vi "IMUOpen.vi"(4 "MagCal":bool=TRUE, 5 "Accel Set":T4={"Data Rate"=enum."1.344 kHz", "Range"=0, "HPF Enable"=FALSE, "HPCF"=enum."00", "Sense Enable"=TRUE, "Accel Scale"={"Xscale"=1.0, "Yscale"=1.0, "Zscale"=1.0}, "Motion Thresh"=0.0} {"Range" items=["+/- 2 G", "+/- 4 G", "+/- 8 G", "+/- 16 G"]}, 6 "Mag Set":T2={"Data Rate"=enum."220 Hz", "Range"=1, "Sense Enable"=TRUE, "Mag Scale"={"Xscale"=1.0, "Yscale"=1.0, "Zscale"=1.0}, "Mag Offset"={"Xzero"=0.0, "Yzero"=0.0, "Zzero"=0.0}, "Anomaly Thresh"=0.0, "Local Mag"=0.0} {"Range" items=["+/- 130 uT"=1, "+/- 190 uT"=2, "+/- 250 uT"=3, "+/- 400 uT"=4, "+/- 470 uT"=5, "+/- 560 uT"=6, "+/- 810 uT"=7]}, 7 "Gyro Set":T5={"Data Rate"=enum."800 Hz", "Range"=0, "HPF Enable"=FALSE, "HPCF"=enum."0000", "Sense Enable"=TRUE} {"Range" items=["+/- 245 deg/sec", "+/- 500 deg/sec", "+/- 2000 deg/sec"]}, 8 "error in (no error)":errorcluster, 9 "Fast":bool=TRUE, 10 "CalSamples":i32=60, 11 "I2C Bus":T3) -> (0 "error out":errorcluster, 2 "Cal Result":T1, 3 "AdaIMUDevRef Out":T6={"DevStatus"={"status"=FALSE, "code"=0, "source"=""}, "Gyro Address"=0, "Gyro Range"=0, "Mean Rates"={"Xmo"=0.0, "Ymo"=0.0, "Zmo"=0.0}, "StdDev Rates"={"Xsdo"=0.0, "Ysdo"=0.0, "Zsdo"=0.0}, "Fast"=FALSE, "Reset"=FALSE, "Accel Address"=0, "Accel Range"=0, "Accel Scale"={"Xscale"=0.0, "Yscale"=0.0, "Zscale"=0.0}, "Mag Address"=0, "Mag Range"=0, "G Sense"=FALSE, "A Sense"=FALSE, "M Sense"=FALSE, "Accel Offset"={"Xzero"=0.0, "Yzero"=0.0, "Zzero"=0.0}, "Motion Thresh"=0.0, "Mag Scale"={"Xscale"=1.0, "Yscale"=1.0, "Zscale"=1.0}, "Mag Offset"={"Xzero"=1.0, "Yzero"=1.0, "Zzero"=1.0}, "I2C Bus"=enum."I2C On-Board", "Handle"=0, "Anomaly Thresh"=0.0, "Local Mag"=0.0})   [LabVIEW 2015]
uses:
  IMUDevRef.ctl
  <vilib>/Rock Robotics/SystemInterfaces/i2clib/i2c_bus.ctl
  <vilib>/Platform/TimedLoop/XDataNode/timing_clust.ctl
  <vilib>/Platform/TimedLoop/XDataNode/nitl_modes.ctl
  <vilib>/Platform/TimedLoop/XDataNode/wakeup.ctl
  <vilib>/Utility/file.llb/Write To Spreadsheet File (DBL).vi
  <vilib>/platform/TimedLoop/XDataNode/XDataNode.xnode
  <vilib>/Platform/TimedLoop/XDataNode/XDNodeRunTimeDep.lvlib
  <vilib>/Analysis/NI_AALBase.lvlib
panel:
  in  "Mag Set 2":T2={"Data Rate"=enum."220 Hz", "Range"=1, "Sense Enable"=TRUE, "Mag Scale"={"Xscale"=1.0, "Yscale"=1.0, "Zscale"=1.0}, "Mag Offset"={"Xzero"=0.0, "Yzero"=0.0, "Zzero"=0.0}, "Anomaly Thresh"=0.0, "Local Mag"=0.0} {"Range" items=["+/- 130 uT"=1, "+/- 190 uT"=2, "+/- 250 uT"=3, "+/- 400 uT"=4, "+/- 470 uT"=5, "+/- 560 uT"=6, "+/- 810 uT"=7]}
  out "XY Mag, Cal'd":cluster{dbl[], dbl[]}(graph)
  out "Anomaly Tol (uT)":dbl
  out "Local Magnitude (uT)":dbl
  out "Mid-Pnt":dbl
  out "Half-Range":dbl
  out "Late?":bool
  in  "Period":i64=20
  out "Yaw":dbl(knob) scale=-180.0..180.0
  out "Pitch":dbl(knob) scale=-90.0..90.0
  out "Roll":dbl(knob) scale=-180.0..180.0
  in  "Reset":bool
  in  "Accel Set 2":T4={"Data Rate"=enum."1.344 kHz", "Range"=0, "HPF Enable"=FALSE, "HPCF"=enum."00", "Sense Enable"=TRUE, "Accel Scale"={"Xscale"=0.9852, "Yscale"=1.0101, "Zscale"=1.0101}, "Motion Thresh"=0.04} {"Range" items=["+/- 2 G", "+/- 4 G", "+/- 8 G", "+/- 16 G"]}
  in  "Gyro Set 2":T5={"Data Rate"=enum."800 Hz", "Range"=0, "HPF Enable"=FALSE, "HPCF"=enum."0000", "Sense Enable"=TRUE} {"Range" items=["+/- 245 deg/sec", "+/- 500 deg/sec", "+/- 2000 deg/sec"]}
  out "Xmagscale":dbl
  out "Ymagscale":dbl
  out "Ymagzero":dbl
  out "Xmagzero":dbl
  out "XY Mag":cluster{dbl[], dbl[]}(graph)
  out "stop loop":bool
  # "EXAMPLE MAGNETOMETER CAL PLOT - FOR REFERENCE"
  # "Magnetometer Cal Results"
  # "Use LM as Local Mag,\nwhich should be NOAA\nHorizontal Mag Intensity.\nUse AT as minimum\nAnomaly Threshold."
  # "Magnetometer Calibration Data Result\n\nLook for a constant radius circle - if not, repeat calibration.\n\nMagnetometer measurement error is generally classified into two categories, Hard Iron and Soft Iron effects.  Only Hard Iron effects\nare compensated here, as they appear more dominate.  Soft Iron effect compensation is a future improvement.  Performance is\nadequate as long as sources of Soft Iron distortion (non-magnetized Iron, Nickle, and Cobalt) are kept away from sensor\n(or vice versa).  If an ellipse is displayed, there is Soft Iron magnetic field interference.  Ensure the cal plot has equally sized X and Y\naxis ranges prior to visually inspecting the cal plot and making an ellipse determination.  If Soft Iron is detected, either relocate the\nIMU or discover and remove the offending material.  Run all motors and other actuators to verify that the Yaw output of the\nComplementary Filter is not significantly affected.  If so, it may be possible to relocate the IMU or shield the motor with\nmu-metal or similar.  Do not shield the IMU!"
  # "Reserved for future use."
  # "These controls/indicators are non-operational / they are here as example documentation only."
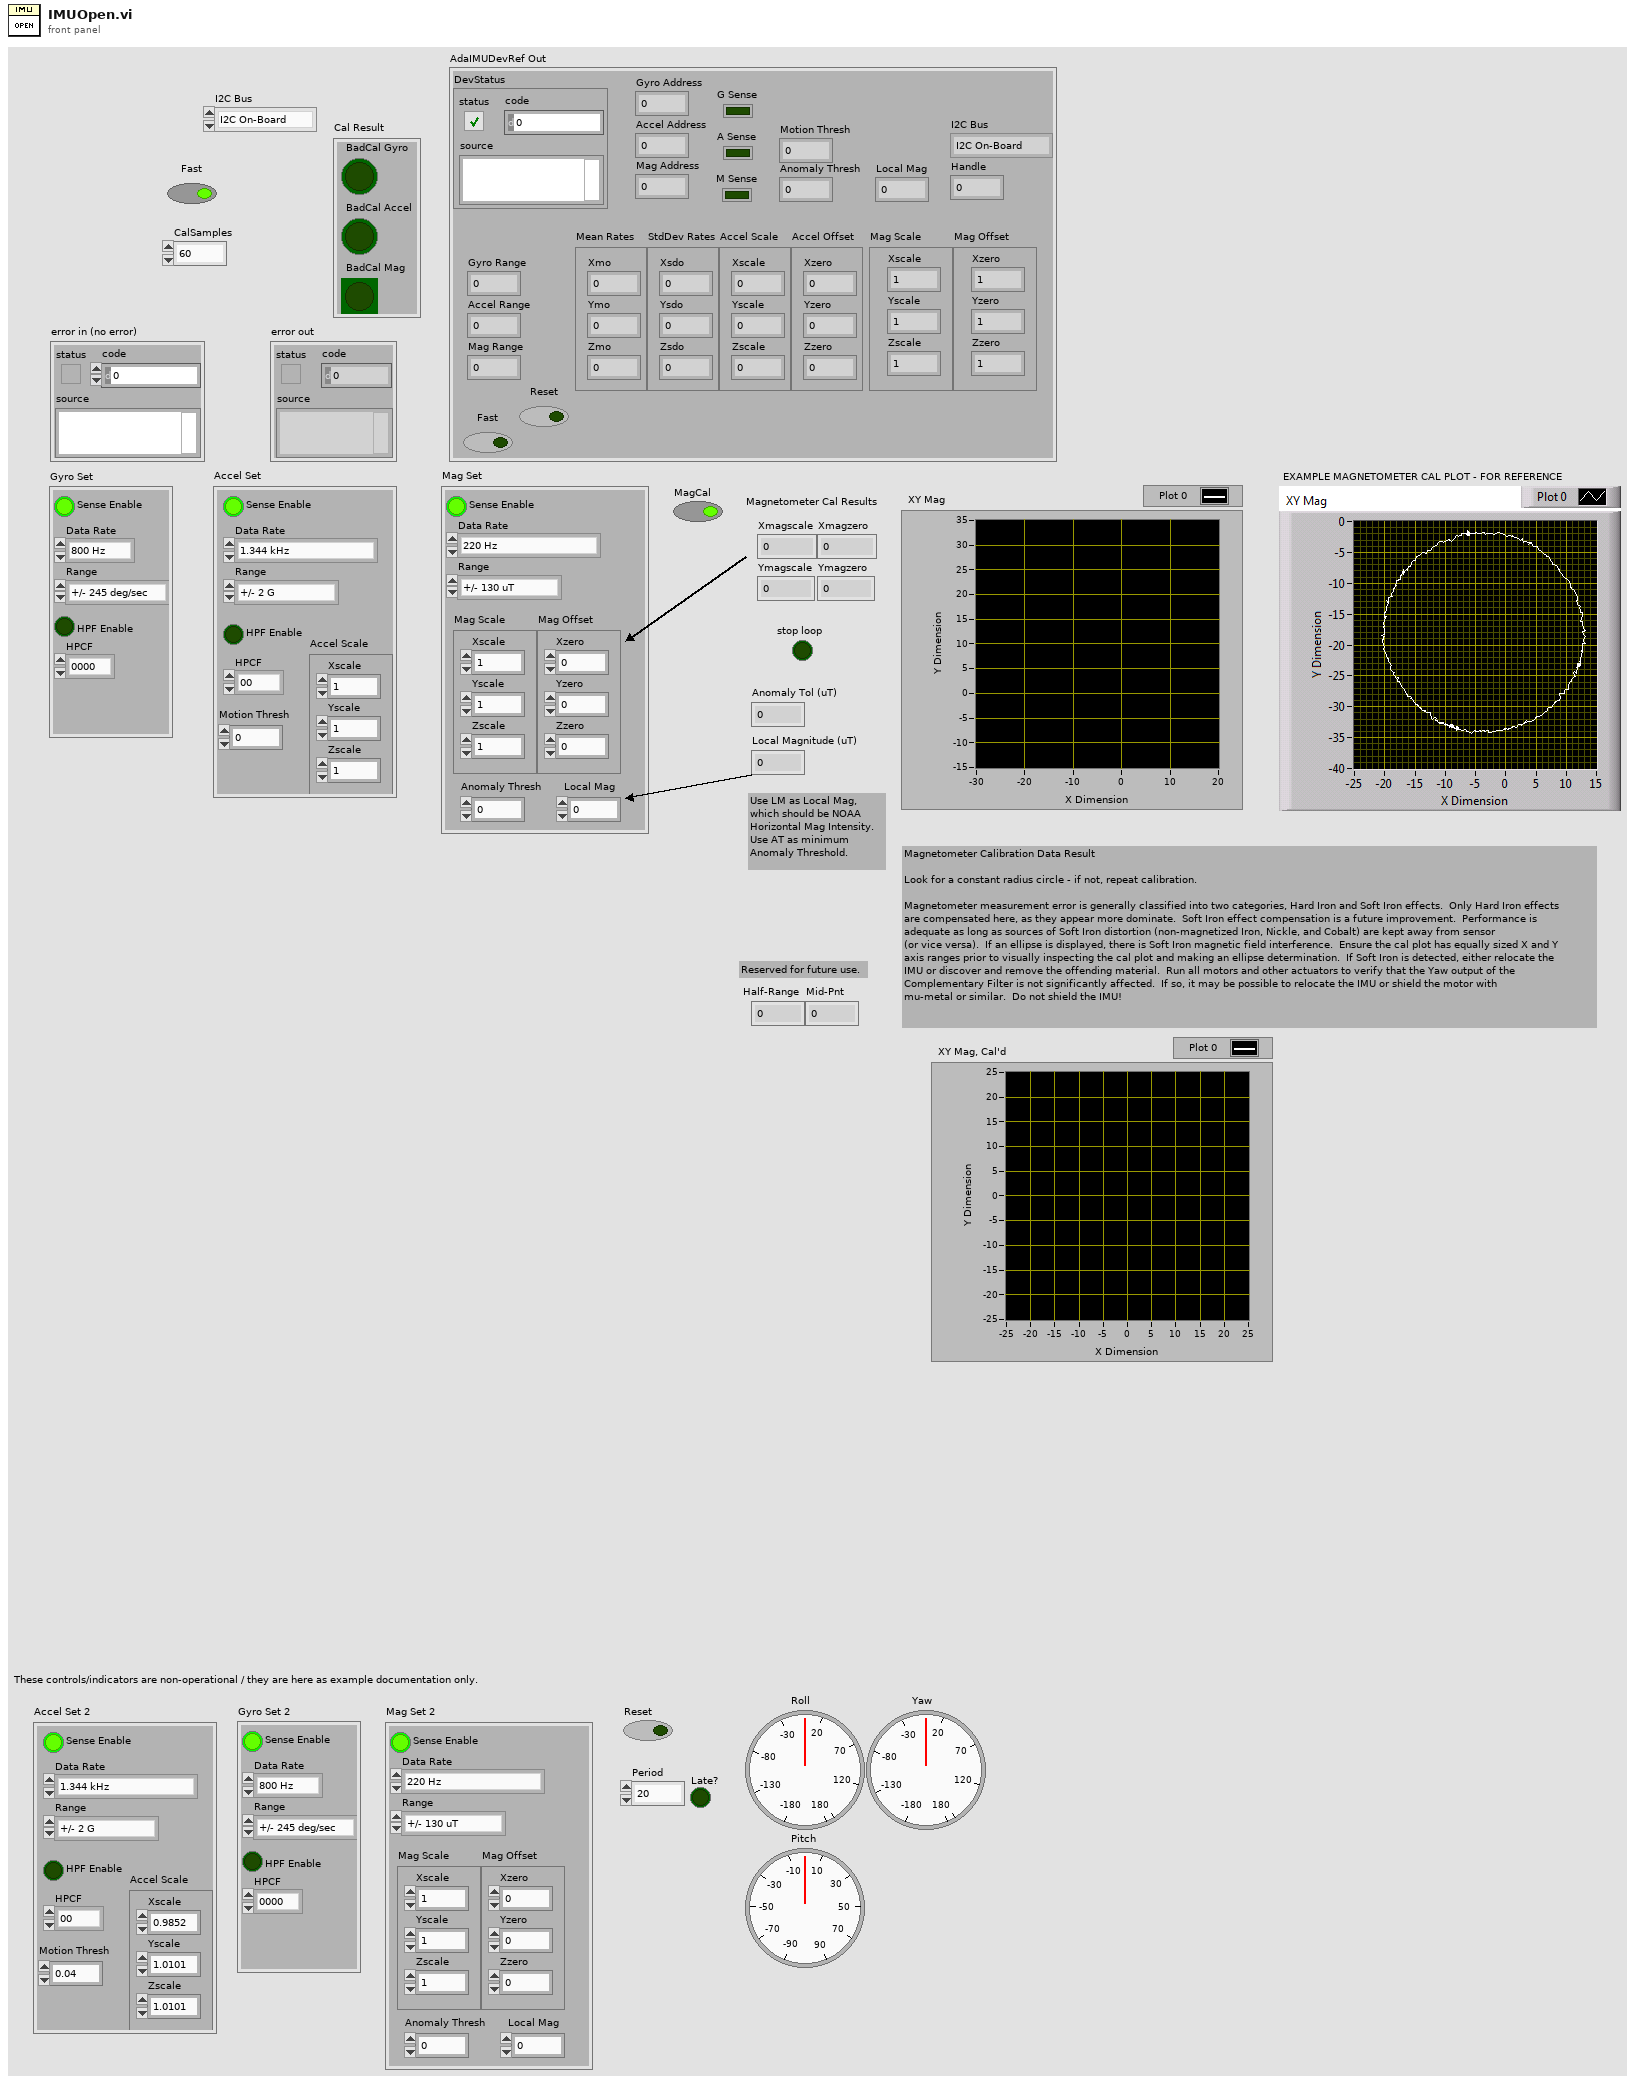
[diagram p1: front panel]
types:
  T1 = cluster{"BadCal Gyro":bool, "BadCal Accel":bool, "BadCal Mag":bool}
  T2 = cluster{"Data Rate":enum8{"0.75 Hz", "1.5 Hz", "3.0 Hz", "7.5 Hz", "15 Hz", "30 Hz", "75 Hz", "220 Hz"}, "Range":u8, "Sense Enable":bool, "Mag Scale":cluster{"Xscale":dbl, "Yscale":dbl, "Zscale":dbl}, "Mag Offset":cluster{"Xzero":dbl, "Yzero":dbl, "Zzero":dbl}, "Anomaly Thresh":dbl, "Local Mag":dbl}
  T3 = typedef "i2c_bus.ctl" = enum16{"I2C On-Board", "I2C MXP", "Invalid"}
  T4 = cluster{"Data Rate":enum8{"Power-down mode", "1 Hz", "10 Hz", "25 Hz", "50 Hz", "100 Hz", "200 Hz", "400 Hz", "Low-power mode only", "1.344 kHz"}, "Range":u8, "HPF Enable":bool, "HPCF":enum8{"00", "01", "10", "11"}, "Sense Enable":bool, "Accel Scale":cluster{"Xscale":dbl, "Yscale":dbl, "Zscale":dbl}, "Motion Thresh":dbl}
  T5 = cluster{"Data Rate":enum8{"100 Hz", "200 Hz", "400 Hz", "800 Hz"}, "Range":u8, "HPF Enable":bool, "HPCF":enum8{"0000", "0001", "0010", "0011", "0100", "0101", "0110", "0111", "1000", "1001"}, "Sense Enable":bool}
  T6 = typedef "IMUDevRef.ctl" = cluster{"DevStatus":errorcluster, "Gyro Address":u8, "Gyro Range":u8, "Mean Rates":cluster{"Xmo":dbl, "Ymo":dbl, "Zmo":dbl}, "StdDev Rates":cluster{"Xsdo":dbl, "Ysdo":dbl, "Zsdo":dbl}, "Fast":bool, "Reset":bool, "Accel Address":u8, "Accel Range":u8, "Accel Scale":cluster{"Xscale":dbl, "Yscale":dbl, "Zscale":dbl}, "Mag Address":u8, "Mag Range":u8, "G Sense":bool, "A Sense":bool, "M Sense":bool, "Accel Offset":cluster{"Xzero":dbl, "Yzero":dbl, "Zzero":dbl}, "Motion Thresh":dbl, "Mag Scale":cluster{"Xscale":dbl, "Yscale":dbl, "Zscale":dbl}, "Mag Offset":cluster{"Xzero":dbl, "Yzero":dbl, "Zzero":dbl}, "I2C Bus":T3, "Handle":i32, "Anomaly Thresh":dbl, "Local Mag":dbl}
  T7 = enum8{"0000", "0001", "0010", "0011", "0100", "0101", "0110", "0111", "1000", "1001"}
  T8 = typedef "WPI_I2CDevRef.ctl" = cluster{"DevStatus":errorcluster, "Device Address":u8, "Handle":i32, "I2C Bus":T3}
  T9 = typedef "XDNodeRunTimeDep.lvlib/timing_clust.ctl" = cluster{"Expected End [f-1]":u64, "Actual End [f-1]":u64, "Finished Late? [f-1]":bool, "Expected End [i-1]":u64, "Actual End [i-1]":u64, "Finished Late? [i-1]":bool, "Expected Start [i]":u64, "Actual Start [i]":u64, "Expected Start [f]":u64, "Actual Start [f]":u64, "Source Name":string, "Structure Name":string, "Period":i64, "Deadline":i64, "Offset":i64, "Start":i64, "Priority":i32, "Timeout":i32, "Mode":T10, "Wakeup Reason":T11, "Error":errorcluster, "Source Type":string, "Secondary Source Type":string, "Global End Time":u64, "Global Start Time":u64, "Frame Duration":u64, "Iteration Duration":u64, "Assigned CPU":i32, "I/O Scan Engine Mode":u32}
  T10 = typedef "XDNodeRunTimeDep.lvlib/nitl_modes.ctl" = enum32{"No Change", "Process missed periods, maintain original phase", "Discard missed periods, maintain original phase", "Process missed periods, ignore original phase", "Discard missed periods, ignore original phase"}
  T11 = typedef "XDNodeRunTimeDep.lvlib/wakeup.ctl" = enum32{"Normal", "Aborted", "Asynchronous wakeup", "Timing source error", "Timed loop error", "Timeout"}
  T12 = typedef "Gyro.ctl" = cluster{"Xrate":dbl, "Yrate":dbl, "Zrate":dbl, "Xdeg":dbl, "Ydeg":dbl, "Zdeg":dbl, "dt":dbl}
  T13 = typedef "Accel.ctl" = cluster{"Xaccel":dbl, "Yaccel":dbl, "Zaccel":dbl, "Motion":bool, "Threshold":dbl, "FreeFall":bool}
  T14 = typedef "Mag.ctl" = cluster{"Xmag":dbl, "Ymag":dbl, "Zmag":dbl, "Anomaly":bool}
  T15 = enum8{"Power-down mode", "1 Hz", "10 Hz", "25 Hz", "50 Hz", "100 Hz", "200 Hz", "400 Hz", "Low-power mode only", "1.344 kHz"}
  T16 = cluster{"Xscale":dbl, "Yscale":dbl, "Zscale":dbl}
  T17 = enum8{"0.75 Hz", "1.5 Hz", "3.0 Hz", "7.5 Hz", "15 Hz", "30 Hz", "75 Hz", "220 Hz"}
  T18 = cluster{"Accel Zero.Zzero":dbl, "Accel Zero.Zzero 2":dbl, "Accel Zero.Zzero 3":dbl}
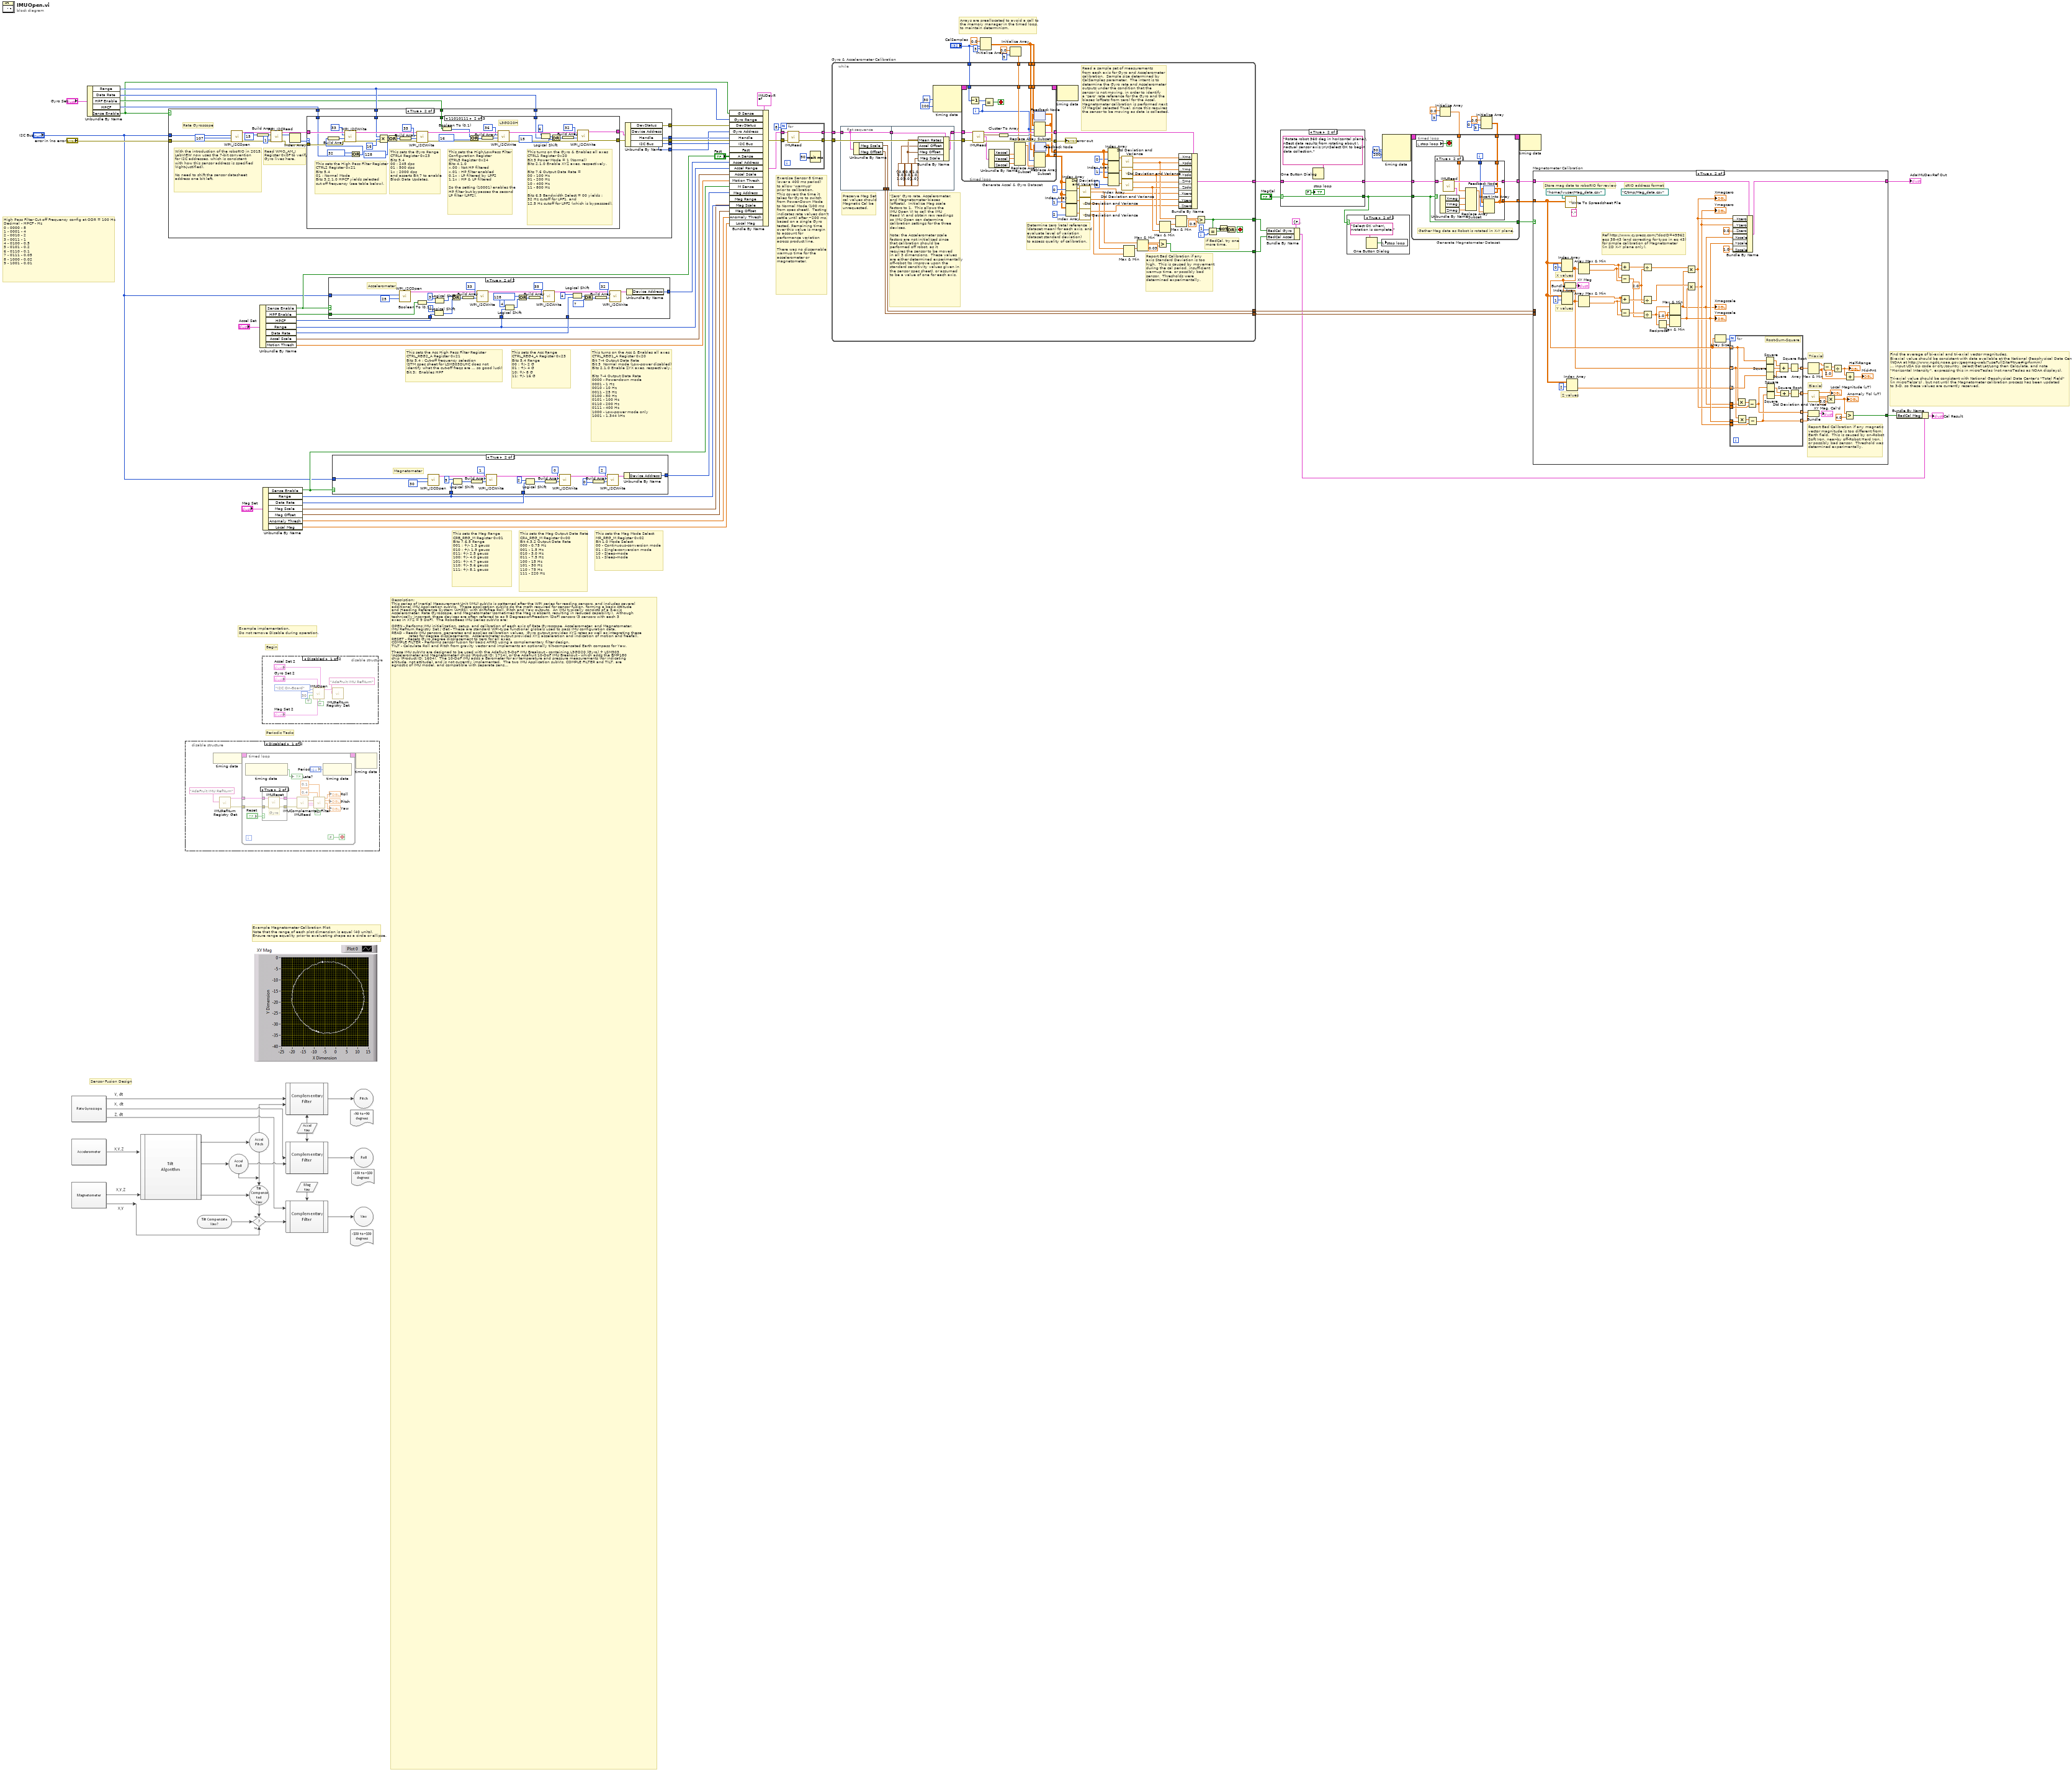
[diagram p0: block diagram]
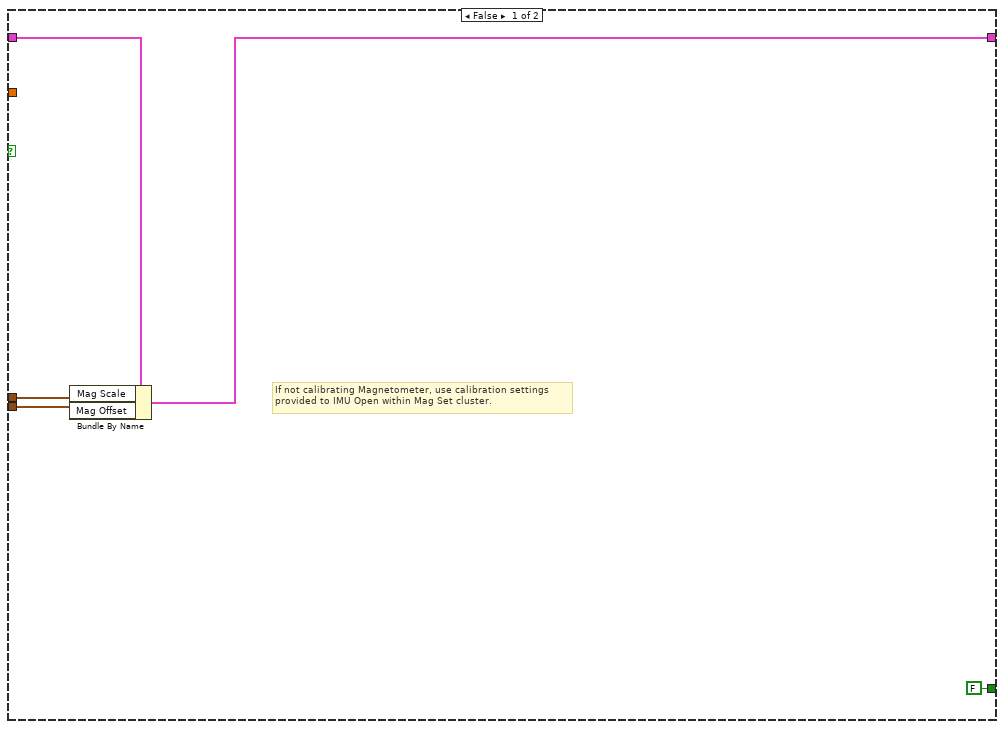
[diagram p2: hidden frame]
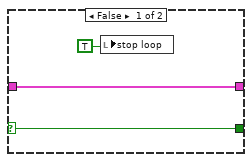
[diagram p5: hidden frame]
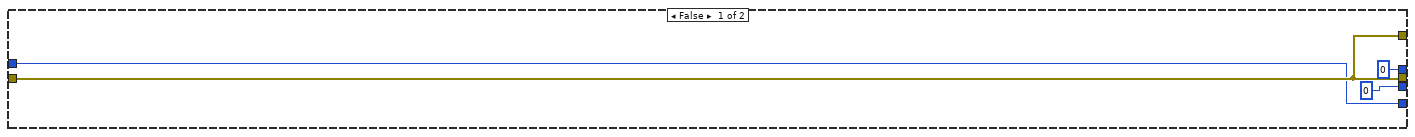
[diagram p9: hidden frame]
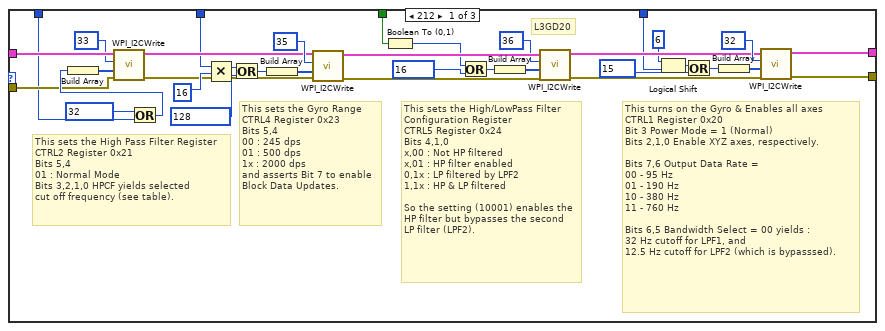
[diagram p10: hidden frame]
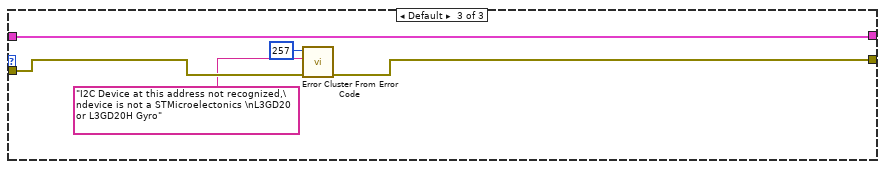
[diagram p11: hidden frame]
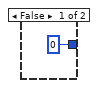
[diagram p12: hidden frame]
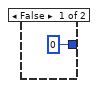
[diagram p13: hidden frame]
diagram:
  # "Find the average of bi-axial and tri-axial vector magnitudes.\nBi-axial value should be consistent with data available at the National Geophysical Data Center\n(NOAA at http://www.ngdc.noaa.gov/geomag-web/?useFullSite=true#igrfwmm)\n... input USA zip code or city/country, select Get Lat/Long then Calculate, and note\n\"Horizontal Intensity\", expressing this in microTeslas (not nanoTeslas as NOAA displays). \n\nTri-axial value should be consistent with National Geophysical Data Center's \"Total Field\"\n(in microTelsa's) , but not until the Magnetometer calibration process has been updated\nto 3-D, so these values are currently reserved."
  # "Arrays are preallocated to avoid a call to\nthe memory manager in the timed loop,\nto maintain determinism."
  # "Sensor Fusion Design"
  # "Example Magnetometer Calibration Plot\nNote that the range of each plot dimension is equal (40 units).\nEnsure range equality prior to evaluating shape as a circle or ellipse."
  # "Begin"
  # "Periodic Tasks"
  # "Example implementation.\nDo not remove Disable during operation."
  # "Description:\nThis series of Inertial Measurement Unit (IMU) subVIs is patterned after the WPI series for reading sensors, and includes several\nadditional IMU Application subVIs.  These application subVIs do the math required for sensor fusion, forming a basic Attitude\nand Heading Reference System (AHRS), with drift-free Roll, Pitch and Yaw outputs.  An IMU typically consists of a 3-axis \nAccelerometer, Rate Gyroscope, and Magnetometer (sometimes the Mag is absent, resulting in reduced capability).  Although\ntechnically incorrect, these devices are often referred to as 9 Degrees-of-Freedom (DoF) sensors (3 sensors with each 3\naxes in XYZ = 9 DoF).  The RoboBees IMU Series subVIs are:\n\nOPEN - Performs IMU initialization, setup, and calibration of each axis of Rate Gyroscope, Accelerometer, and Magnetometer.\nIMU RefNum Registry Set / Get - These are standard WPI-type functional globals used to pass IMU configuration data.\nREAD - Reads IMU sensors, generates and applies calibration values.  Gyro output provides XYZ rates as well as integrating these\n              rates for degree displacements.  Accelerometer output provides XYZ acceleration and indication of motion and freefall.\nRESET - Resets Gyro degree displacement to zero for all axes.\nCOMPLE FILTER - Performs sensor fusion for basic AHRS using a complementary filter design.\nTILT - Calculate Roll and Pitch from gravity vector and implements an optionally tilt-compensated Earth compass for Yaw.\n\nThese IMU subVIs are designed to be used with the Adafruit 9-DoF IMU Breakout - containing L3GD20 (Gyro) + LSM303 \n(Accelerometer and Magnetometer) chips (Product ID: 1714), or the Adafruit 10-DoF IMU Breakout - which adds the BMP180\nchip (Product ID: 1604).  The 10-DoF IMU adds a Barometer for air temperature and pressure measurements (for indicating\naltitude, not attitude), and is not currently implemented.  The two IMU Application subVIs, COMPLE FILTER and TILT, are\nagnostic of IMU model, and compatible with separate sensors, as long as all sensor axes are aligned properly.\n\nThe motivation to fusing these sensors is to combine their best properties and mitigate the worst properties of each.  The overall\nsensor fusion design is provided (to lower left) in block diagram form.  A major benefit is effective elimination of the drift inherent\nin the Rate Gyro when used alone.\n\nDesign:\nThe IMU OPEN subVI sets up each sensor based on the respective Set Cluster settings.  This includes setting the sensor range, output\ndata rate, enabling the High Pass Filter (Gyro and Accelerometer only), and selecting a High Pass Cut off Frequency.  Each sensor\ncan also be selectively enabled/disabled.  All sensors (except the Barometer), need to be enabled for a fully functional AHRS.  The\nIMU breakout board from Adafruit.com places all sensors on a common I2C bus for communication.  The sensor chip's I2C\nAddresses (in hex) and respective data sheets for I2C register references are:\n\nChip                      -  Sensor                - I2C Address  -  Data Sheet Reference\nLSM303DLHC      - Accelerometer   - 0x19               -  http://www.adafruit.com/datasheets/LSM303DLHC.PDF\nLSM303DLHC      - Magnetometer  - 0x1E               -  see above\nL3GD20(H)           - Rate Gyroscope - 0x6B               -  http://www.st.com/st-web-ui/static/active/en/resource/technical/document/\n                                                                                          datasheet/DM00036465.pdf\nBMP180               - Barometer           - 0x77               -  http://www.adafruit.com/datasheets/BST-BMP180-DS000-09.pdf\n\nNote: Adafruit modified both breakout board configurations in Oct of 2014 to upgrade the Gyro sensor from L3GD20 to L3GD20H\n(improved performance specifications).  This code should be compatible with each Gyro variant.  Guidance on the Gyro startup\nsequence is given in section 3.1 of ST MicroElectronics App Note AN4506 for L3GD20H : \nhttp://www.st.com/web/en/resource/technical/document/application_note/DM00119037.pdf\n\nAfter the sensors are set up, enabled sensors are turned on, IMU configuration data is loaded into an IMU Cluster, and sensor\ncalibration begins.\n\nCalibration:\nRaw readings from an IMU are not very useful until they are conditioned by carefully determined calibration parameters.\nSince reading the digital sensor values is a bit complicated, the IMU READ subVI is simply called by IMU OPEN to produce the raw\nmeasurement values used to characterize the sensor.  The calibration is only good for the range selected during the cal process.\n\nThe calibration process used here is determining the values 'm' and 'b' for the assumed linear sensor model Y=mX+b for each\nparameter/axis pair, where 'X' is the raw sensor reading, 'm' and 'b' are cal parameters, and 'Y' is the corrected sensor reading.\nThe sensor is 'exercised' eight times to allow the Gyro readings to reach steady-state, which improves the calibration.  With the\ndefault cal sample size of 60, the Gyro/Accelerometer cal process takes about 2.2 seconds, which is about 0.2 seconds longer\nthan the default cal time for the OPEN subVI for an analog Gyro.   The Gyro and Accelerometer cal is performed first\n(simultaneously), and the robot needs to be completely still during this time (as is required with an analog Gyro).  Since the cal\nis conducted within the OPEN subVI, and OPEN is generally placed in Begin (in FIRST Robotics) before the robot can move itself,\nthis requirement is easily fulfilled.  Care, however, must still be taken to ensure no external bumps occur during this cal.  This\ncode can actually detect if a physical disturbance occurred, and recalibrate automatically as a mitigation (no extra charge).\n\nRecalling the model Y=mX+b, for the IMU Gyro, 'm' is taken from the spec sheet as the gain (sensitivity) for each axis.  Value 'b',\nwhich is bias from zero, is determined by taking the statistical mean of a sample of Gyro rate measurements while the sensor is still.\n\nFor the Accelerometer, 'm' should be determined off-robot, as it requires the sensor to be moved in all 3 dimensions.  These values\nare either determined experimentally off-robot (to improve upon the standard sensitivity values given in the sensor spec sheet), or\nassumed to be a value of one for each axis.  To determine experimentally, find the maximum and minimum values of each axis as\nthey are rotated (slowly) through vertical.  The axis sensitivity is half of the signed difference between max and min.  Value 'b' is\ndetermined automatically by taking the statistical mean of a sample of Accelerometer measurements while the sensor is still.\n\nThe fun really begins with the Magnetometer calibration.  Proper Mag cal requires the sensor to be rotated in all 3 dimensions, but\nunlike the Accelerometer, the Mag must be rotated with the rest of the robot to account for how the robot itself disturbs the Earth's\nmagnetic field (this is a lot easier when the Mag sensor is installed in a smart phone.).  Since one typically would not have available\na 3-axis non-ferrous robot gimbal, the cal process is designed to support a 2-D calibration in the X-Y (horizontal) plane only.\n\nIn another departure from the Gyro/Accel cal, sample data from the Mag must be taken as the robot is moving.  This process is\noptional to allow the 'm' and 'b' Mag cal parameters to be determined during final testing, and then loaded into the Mag Set Cluster\nfor operations (i.e. competition).  If selected, the Mag cal process first instructs you to begin rotating the robot (manually) with a \npop-up dialog box.  Selecting OK initiates data collection, and provides a second dialog box to allow you to signal when you've \ncompleted a 360 degree rotation.  \n\nOnce complete, the X and Y axis 'm' and 'b' parameters are calculated and displayed on the IMU OPEN Front Panel as 'scale' and\n'zero', respectively.  An XY graph of the data is also provided to allow visual inspection of the cal result - look for a nicely shaped\ncircle (see example at left), if not, repeat the cal.  If you like the plot, load the X and Y axis scale and zero parameters into the Mag\nSet Cluster, retain the default scale (1) and zero (0) values for the Mag Z axis, and turn off Mag cal by deasserting MagCal.\n\nMagnetometer measurement error is generally classified into two categories, Hard Iron and Soft Iron effects.  Only Hard Iron effects\nare compensated here, as they appear to dominate.  Soft Iron effect compensation is a future improvement.  Performance is\nadequate as long as sources of Soft Iron distortion (non-magnetized Iron, Nickle, and Cobalt) are kept away from sensor\n(or vice versa).  If an ellipse is displayed, there is Soft Iron magnetic field interference.  Ensure the cal plot has equally sized X and Y\naxis ranges prior to visually inspecting the cal plot and making an ellipse determination.  If Soft Iron is detected, either relocate the\nIMU or discover and remove the offending material.  Run all motors and other actuators to verify that the Yaw output of the\nComplementary Filter is not significantly affected.  If so, it may be possible to relocate the IMU or shield the motor with\nmu-metal or similar.  Do not shield the IMU!\n\nInputs:\nDIO MODULE - Digital Module designation.\nCALSAMPLES - Number of samples taken for Gyro and Accelerometer calibration process.\nFAST - Boolean, if True, bypasses sensor data ready status verification in the interest of faster IMU Read operations.\n             Setting this to False will force each sensor to verify that data is ready prior to an IMU Read.\nMAGCAL - Boolean, if True, activates the Magnetometer calibration process within IMU OPEN.\n                    Setting this to False skips the Mag cal process, applying cal parameters defined in the Mag Set Cluster during IMU Read.\nGYRO SET -\n     SENSE ENABLE - Enables the Gyro Sensor when True, allowing OPEN IMU to set up and turn on the Gyro, and READ IMU to read. \n                                   Setting this to False speeds up the IMU READ operation, should this sensor not be required.\n     DATA RATE - Sets the sensor output data rate in Hertz. \n     RANGE - Sets the sensor range, in degrees / second.\n     HPF ENABLE - Enables the Gyro High Pass Filter when True. \n     HPCF - Sets the High Pass Cut off Frequency.  Values are specific enumerated binary nybbles that correspond to cut off\n                   frequencies in Hertz.  See Table (near code) for selections at 100 Hz data rate.  See spec sheet for additional detail.\nACCEL SET - \n     SENSE ENABLE -  Enables the Accel Sensor when True, allowing OPEN IMU to set up and turn on the Accel, and READ IMU to read.\n                                    Setting this to False speeds up the IMU READ operation, should this sensor not be required. \n     DATA RATE - Sets the sensor output data rate in Hertz.\n     RANGE - Sets the sensor range, in G's (1 G is ~ 9.805 meters / second^2).  The Earth's gravity field is, well, about 1 G at sea level.\n     HPF ENABLE - Enables the Accelerometer High Pass Filter when True. \n     HPCF - Sets the High Pass Cut off Frequency.  Values are specific enumerated bit pairs that correspond to cut off frequencies in\n                   Hertz.  Spec sheet does not define to what cut off frequencies these settings correspond.  Suggest experiment.\n     ACCEL SCALE - Multiplier value for each axis to correct for imperfection in spec sheet cal factors. \n     MOTION THRESH - Threshold value used to signal the detection of Motion or Free Fall, specified in G's. \nMAG SET - \n     SENSE ENABLE -  Enables the Mag Sensor when True, allowing OPEN IMU to set up and turn on the Mag, and READ IMU to read.\n                                   Setting this to False speeds up the IMU READ operation, should this sensor not be required. \n     DATA RATE - Sets the sensor output data rate in Hertz.\n     RANGE - Sets the sensor range, in microTesla's (1 uT = 0.01 Gauss).  The Earth's magnetic field (magnitude) is about 0.5 Gauss,\n                     or ~50 uT, with both horizontal (North and East) and vertical (Down) components that change with locale (and time). \n     MAG SCALE -  Multiplier value to correct raw Magnetometer reading to calibrated value.  Calculated by the Mag cal process.\n     MAG OFFSET - Offset value to correct raw Magnetometer reading to calibrated value.  Calculated by the Mag cal process.\n     ANOMALY THRESH - Threshold value used to signal the detection of a magnetic anomoly, i.e. a disturbance in the Earth field,\n                                            specified in uTeslas.\n     LOCAL MAG - Bi-axial horizontal vector magnitude of local Earth's magnetic field, specified in uTeslas.\n     \nOutputs:\nADAIMUDEVREF OUT - Device Reference containing IMU configuration data. \nBADCAL GYRO - Boolean, if True, indicates excessive variation in sample data set.  Likely Gyro moved during cal process.  If True,\n                              Gyro cal process will automatically repeat one additional time in an attempt to recover.\n                              If False, sample data set variation low enough to indicate Gyro was still during cal, and zero-rate mean is trusted. \nBADCAL ACCEL - Boolean, if True, indicates excessive variation in sample data set.  Likely Accel moved during cal process.\n                              If False, sample data set variation low enough to indicate Accel was still during cal, and mean is trusted as the bias.\nBADCAL MAG - Boolean, if True, indicates excessive variation in the magnetic field as measured during calibration.  Possible causes\n                             are nearby hard iron off-robot, soft iron on-robot, or poor rotation during calibration.\n\nFuture Improvements:\nBarometer, move freefall into interrupt/DIO, DCM/Kalman filter, Soft Iron Calibration, 3D cal, Auto ranging, FPGA integration,\nFuse Mag-based Yaw with differential encoders to correct for external-to-robot ferrous sources, SPI interface for faster read response,\nCal status VI\n\nVI Properties:\nExecution Reentrancy is set to Non Reentrant Execution\n\nImplementation:\nCode as per example on upper left.  Experimentally determine values for Accelerometer scale as described in above section on\ncalibration, and load into the Accel Set Cluster (or default to one).  Set appropriate ranges, fastest data rates (if polling), and enable\neach sensor. Install sensor on robot and initially set MagCal to True.  Determine Mag cal parameters as described above and load\nthese values into Mag Set Cluster.  Set MagCal to False to skip future Mag cals.\n\nMagnetic Anomalies are detected during IMU READ operation by comparing the root-sum-square of the X-Y axes to the horizontal\nmagnitude of the local Earth field, based on two settings which must be specified in the IMU OPEN Mag Set Cluster.  The first setting\nis LOCAL MAG, representing the biaxial horizontal vector magnitude of the Earth's local magnetic field.  This can be found from data\navailable at the National Geophysical Data Center, part of the National Oceanic and Atmospheric Administration (NOAA) at :\n\nhttp://www.ngdc.noaa.gov/geomag-web/?useFullSite=true#igrfwmm\n\nTo find the value for LOCAL MAG, input USA zip code or city/country, select Get Lat/Long then Calculate, and use the \"Horizontal Intensity\"\nvalue for Local Mag, expressing this in uTeslas (not nTeslas as NOAA displays), or use the calculated value \"Local Magnitude (uT)\" produced\nby this VI (under Magnetometer Cal Results).  The second setting is ANOMALY THRESH, also specified in the Mag Set Cluster, and is used as\ntolerance for the comparison.  Set to a value at least as large as \"Anomaly Tol (uT)\", also produced by this VI.  Based on these settings,\nIMU READ produces a Boolean Magnetic Anomaly indication that can be used to determine when the Magnetometer is reading more than\nthe Earth's field. In this situation, the Yaw output of the sensor fusion Complementary Filter should not be trusted to be accurate.\n\nThe anomaly threshold can be increased above the value reported as Anomaly Tol (uT) to avoid false positive indications, but this is at the\nexpense of reduced sensitivity to actual magnetic anomalies.  Ideally, detection of a Magnetic Anomaly should occur before the Yaw\nreading is substantially affected.  This may be difficult to achieve without very careful calibration of the Mag, and careful selection of the\nanomaly threshold.  \n \nThe Mag cal values are strongly a function of where the sensor is located on the robot, and what is installed nearby, so it's important\nto recalibrate fairly often, certainly after relocating the sensor, and again after the robot is completely assembled.  Be sure you actuate\nall motors and mechanisms to test for interaction with the Yaw indication, which uses the Mag.  Be aware that another robot that\ncomes close to the Magnetometer might disturb the local magnetic field enough to cause error in Yaw - the solution to this difficulty\nis left to the enterprising student of sensor fusion.\n\nEnabling the Gyro and Accelerometer High Pass Filters (HPF) can have a deleterious effect on dynamic response, as they can\nintroduce lag.  HPFs default to off, but advanced control system designers may find them useful.  Experiment cautiously.\n\nThe Accelerometer senses both gravitation and accelerating movement (study Einstein's principle of Equivalence).  Roll and Pitch may be\naffected by movement, as will Yaw should Tilt-Compensation be enabled (this is selected with the Comple Filter subVI).\n\nConfiguring these IMU subVIs per the example creates a simple Attitude and Heading Reference System (AHRS).  The range of Pitch/\nRoll/Yaw values are constrained in range, however, as follows:  Pitch range is -90<P<+90, Roll range is -180<R<+180, and Yaw range\nis -180<Y<+180.  Although over-rotating Pitch and Yaw beyond their range will result in erroneous readings, this should be an\nadequate operating range for most robot body applications.  These range constraints may or may not be adequate for an actuator\nor mechanism.  Yaw is a bit different ...  North is 0 degrees, and East/West  is -90/+90 deg, respectively.  South is both -180 and +180\ndeg, as these values are congruent.  It is ok to over-rotate Yaw, as this portion of the Complementary Filter is designed with logic to\nsmoothly transition across the +/-180 degree discontinuity (auto-wrap).\n \nIt is important to note that while the P/R/Y values are constrained, the Gyro displacement values in X/Y/Z are not.  Gyro deg outputs\nfrom the IMU READ subVI will wind (not wrap) - i.e. they will continue to count above/below 360 degrees.  Use the LabVIEW\nQuotient & Remainder (modulus) function to convert these outputs to a wrapping behavior, if desired. \n\nImplementation considerations for IMU Read:\nThis design performs numerical integration off-FPGA for the Digital Gyro (unlike the Analog Gyro subVIs, which typically utilize\nthe FPGA to perform accumulation for superior speed resulting in less integration error).   Testing indicates this off-FPGA\napproach may be adequate for FRC application, however, it is important to ensure the code runs without any timing issues.\nThis is why a Timed Loop is recommended for the IMU Read within Periodic Tasks (executes at a higher priority).  Non-uniformity\nin read iteration is mitigated by design, as each dt is uniquely calculated by time stamping each read event.  This means that while\nsome variation in timing can be tolerated (the occasional late iteration), excessively long durations (periods) between successive\nreads will fail to capture the actual rate profile as it changes resulting in integration error.  \n\nIn short, use a Timed Loop structure to iterate IMU READs, and set the loop period for a relatively fast iteration (<75 ms).  Shorter\nperiods provide improved accuracy of degree displacements, however setting this too short can impact the execution of your\nremaining code (especially when using Timed Loops).  One way of determining an optimized period is to set it while monitoring\nthe \"Finished Late?\" Loop parameter, ensuring this value stays False.   It helps if the CPU Utilization remains low (<75%), which\ncan be monitored with the RT Get CPU Loads subVI (Real Time menu).  Study LabVIEW determinism for additional insight.\n\n----- RoboBees FRC Team 836! -----  You too can conquer inertia!! ... consider a career in STEM!"
  # "This sets the Mag Mode Select\nMR_REG_M Register 0x02\nBit 1,0 Mode Select\n00 - Continuous-conversion mode \n01 - Single-conversion mode\n10 - Sleep-mode\n11 - Sleep-mode"
  # "This sets the Mag Output Data Rate\nCRA_REG_M Register 0x00\nBit 4,3,2 Output Data Rate\n000 - 0.75 Hz \n001 - 1.5 Hz \n010 - 3.0 Hz\n011 - 7.5 Hz\n100 - 15 Hz\n101 - 30 Hz\n110 - 75 Hz\n111 - 220 Hz"
  # "This sets the Mag Range\nCRB_REG_M Register 0x01\nBits 7,6,5 Range\n001 : +/- 1.3 gauss\n010 : +/- 1.9 gauss\n011: +/- 2.5 gauss\n100: +/- 4.0 gauss\n101: +/- 4.7 gauss\n110: +/- 5.6 gauss\n111: +/- 8.1 gauss"
  # "This sets the Acc Range\nCTRL_REG4_A Register 0x23\nBits 5,4 Range\n00 : +/- 2 G\n01 : +/- 4 G\n10: +/- 8 G\n11: +/- 16 G"
  # "This turns on the Acc & Enables all axes\nCTRL_REG1_A Register 0x20\nBit 7-4 Output Data Rate\nBit 3  Normal mode (Low-power disabled)\nBits 2,1,0 Enable ZYX axes, respectively.\n\nBits 7-4 Output Data Rate \n0000 - Power-down mode\n0001 - 1 Hz \n0010 - 10 Hz\n0011 - 25 Hz\n0100 - 50 Hz\n0101 - 100 Hz\n0110 - 200 Hz\n0111 - 400 Hz\n1000 - Low-power mode only\n1001 - 1.344 kHz"
  # "This sets the Acc High Pass Filter Register\nCTRL_REG2_A Register 0x21\nBits 5,4 : Cut-off frequency selection\n(STM spec sheet for LSM303DLHC does not\nidentify what the cut-off freqs are ... so good luck)\nBit 3:  Enables HPF"
  # "High Pass Filter Cut off Frequency config at ODR = 100 Hz\nDecimal\t-\tHPCF\t-\tHz\n0\t-\t0000\t-\t8\n1\t-\t0001\t-\t4\n2\t-\t0010\t-\t2\n3\t-\t0011\t-\t1\n4\t-\t0100\t-\t0.5\n5\t-\t0101\t- 0.2\n6\t-\t0110\t-\t0.1\n7\t-\t0111\t-\t0.05\n8\t-\t1000\t-\t0.02\n9\t-\t1001\t-\t0.01"
  # "Exercise Sensor 8 times\n(over a 400 ms period)\nto allow 'warmup'\nprior to calibration.\nThis covers the time it\ntakes for Gyro to switch\nfrom Power-Down Mode\nto Normal Mode (100 ms\nfrom spec sheet).  Testing\nindicates rate values don't\nsettle until after ~200 ms,\nbased on a single Gyro\ntested. Remaining time\nover this value is margin\nto account for\nperformance variation\nacross product line.\n\nThere was no discernable\nwarmup time for the\naccelerometer or\nmagnetometer."
  n1 = Unbundle By Name("Gyro Set") -> ("Range"=w61:u8, "Data Rate"=w60:enum8{"100 Hz", "200 Hz", "400 Hz", "800 Hz"}, "HPF Enable"=w59:bool, "HPCF"=w58:T7, "Sense Enable"=w51:bool)
  n2 = case shown="True" w51 {
    tunnel: "error in (no error)" -> [w75 w97]
    tunnel: [w75 w86] -> w69
    tunnel: [u8 0 ("Device Address") w85] -> w68
    tunnel: [w75 w84] -> w46
    tunnel: w61 -> [_ w83]
    tunnel: w60 -> [_ w82]
    tunnel: w59 -> [_ w81]
    tunnel: w58 -> [_ w80]
    tunnel: "I2C Bus" -> [w72 w79]
    tunnel: [0 ("Handle") w78] -> w41
    tunnel: [w72 w77] -> w42
    frame False {
    }
    frame True {
      # "Rate Gyroscope"
      # "Read WHO_AM_I \nRegister 0x0F to verify\nGyro lives here."
      # "With the introduction of the roboRIO in 2015,\nLabVIEW now uses the 7-bit convention\nfor I2C addresses, which is consistent\nwith how this sensor address is specified\n(right-justified).\n\nNo need to shift the sensor datasheet\naddress one bit left."
      n3 = call <vilib>:"WPI_I2COpen.vi"("error in"=w97, "Device Address"=u8 107 ("Data To Send"), "I2C Bus"=w79) -> ("error out"=w93:errorcluster, "I2CDevRef"=w88:T8)  [unwired: 7 in]
      n4 = Build Array(u8 15 ("Data To Send")) -> (w95:u8[])
      n5 = call <vilib>:"WPI_I2CRead.vi"("error in (no error)"=w93, "I2CBytesToRead"=u8 1, "I2CRegister"=w95, "I2CDevRef"=w88) -> ("error out"=w90:errorcluster, "Data Out"=w92:u8[], "I2CDevRef"=w89:T8)  [unwired: 5 in]
      n6 = Index Array(array=w92) -> (element=w91:u8)  [unwired: 1 in]
      n7 = case shown="11010111" w91 {
        tunnel: [w132 w167 w172] -> w87
        tunnel: [w131 w166 w168] -> w84
        tunnel: w89 -> [w130 w165 w172]
        tunnel: w90 -> [w115 w151 w171]
        tunnel: w83 -> [w111 w147 _]
        tunnel: w80 -> [w110 w146 _]
        tunnel: w81 -> [w105 w141 _]
        tunnel: w82 -> [w101 w135 _]
        frame 212 {
          # "L3GD20"
          # "This sets the High Pass Filter Register\nCTRL2 Register 0x21\nBits 5,4\n01 : Normal Mode\nBits 3,2,1,0 HPCF yields selected\ncut off frequency (see table)."
          # "This sets the High/LowPass Filter\nConfiguration Register\nCTRL5 Register 0x24\nBits 4,1,0  \nx,00 : Not HP filtered\nx,01 : HP filter enabled\n0,1x : LP filtered by LPF2\n1,1x : HP & LP filtered\n\nSo the setting (10001) enables the\nHP filter but bypasses the second\nLP filter (LPF2)."
          # "This sets the Gyro Range\nCTRL4 Register 0x23\nBits 5,4\n00 : 245 dps\n01 : 500 dps\n1x : 2000 dps\nand asserts Bit 7 to enable Block Data Updates."
          # "This turns on the Gyro & Enables all axes\nCTRL1 Register 0x20\nBit 3 Power Mode = 1 (Normal)\nBits 2,1,0 Enable XYZ axes, respectively.\n\nBits 7,6 Output Data Rate = \n00 - 95 Hz\n01 - 190 Hz \n10 - 380 Hz\n11 - 760 Hz\n\nBits 6,5 Bandwidth Select = 00 yields : \n32 Hz cutoff for LPF1, and\n12.5 Hz cutoff for LPF2 (which is bypasssed)."
          n8 = Or(x=u8 32 ("Data To Send"), y=w110) -> (x .or. y?=w120:u8)
          n9 = Build Array(w120) -> (w123:u8[])
          n10 = call <vilib>:"WPI_I2CWrite.vi"("error in (no error)"=w115, "I2CDataToSend"=w123, "I2CRegister"=u8 33 ("Data To Send"), "I2CDevRef"=w130) -> ("error out"=w114:errorcluster, "I2CDevRef"=w122:T8)  [unwired: 6 in]
          n11 = Multiply(x=w111, y=u8 16) -> (x*y=w109:u8)
          n12 = Or(x=w109, y=u8 128 ("Data To Send")) -> (x .or. y?=w108:u8)
          n13 = Build Array(w108) -> (w127:u8[])
          n14 = call <vilib>:"WPI_I2CWrite.vi"("error in (no error)"=w114, "I2CDataToSend"=w127, "I2CRegister"=u8 35 ("Data To Send"), "I2CDevRef"=w122) -> ("error out"=w113:errorcluster, "I2CDevRef"=w119:T8)  [unwired: 6 in]
          n15 = Boolean To (0,1)(Boolean=w105) -> (0, 1=w99:i16)
          n16 = Or(x=w99, y=u8 16 ("Data To Send")) -> (x .or. y?=w107:i16)
          n17 = Build Array(w107) -> (w116:i16[])
          n18 = call <vilib>:"WPI_I2CWrite.vi"("error in (no error)"=w113, "I2CDataToSend"=w116, "I2CRegister"=u8 36 ("Data To Send"), "I2CDevRef"=w119) -> ("error out"=w112:errorcluster, "I2CDevRef"=w118:T8)  [unwired: 6 in]
          n19 = Logical Shift(y=i16 6, x=w101) -> (x << y=w102:u32)
          n20 = Or(x=w102, y=u8 15 ("Data To Send")) -> (x .or. y?=w104:u32)
          n21 = Build Array(w104) -> (w128:u32[])
          n22 = call <vilib>:"WPI_I2CWrite.vi"("error in (no error)"=w112, "I2CDataToSend"=w128, "I2CRegister"=u8 32 ("Data To Send"), "I2CDevRef"=w118) -> ("error out"=w131:errorcluster, "I2CDevRef"=w132:T8)  [unwired: 6 in]
        }
        frame 215 {
          # "L3GD20H"
          # "This sets the High Pass Filter Register\nCTRL2 Register 0x21\nBits 5,4\n01 : Normal Mode\nBits 3,2,1,0 HPCF yields selected\ncut off frequency (see table below)."
          # "This sets the High/LowPass Filter\nConfiguration Register\nCTRL5 Register 0x24\nBits 4,1,0  \nx,00 : Not HP filtered\nx,01 : HP filter enabled\n0,1x : LP filtered by LPF2\n1,1x : HP & LP filtered\n\nSo the setting (10001) enables the\nHP filter but bypasses the second\nLP filter (LPF2)."
          # "This sets the Gyro Range\nCTRL4 Register 0x23\nBits 5,4\n00 : 245 dps\n01 : 500 dps\n1x : 2000 dps\nand asserts Bit 7 to enable Block Data Updates."
          # "This turns on the Gyro & Enables all axes\nCTRL1 Register 0x20\nBit 3 Power Mode = 1 (Normal)\nBits 2,1,0 Enable XYZ axes, respectively.\n\nBits 7,6 Output Data Rate = \n00 - 100 Hz\n01 - 200 Hz \n10 - 400 Hz\n11 - 800 Hz\n\nBits 6,5 Bandwidth Select = 00 yields : \n32 Hz cutoff for LPF1, and\n12.5 Hz cutoff for LPF2 (which is bypasssed)."
          n23 = Or(x=u8 32 ("Data To Send"), y=w146) -> (x .or. y?=w156:u8)
          n24 = Build Array(w156) -> (w159:u8[])
          n25 = call <vilib>:"WPI_I2CWrite.vi"("error in (no error)"=w151, "I2CDataToSend"=w159, "I2CRegister"=u8 33 ("Data To Send"), "I2CDevRef"=w165) -> ("error out"=w150:errorcluster, "I2CDevRef"=w158:T8)  [unwired: 6 out]
          n26 = Multiply(x=w147, y=u8 16) -> (x*y=w145:u8)
          n27 = Or(x=w145, y=u8 128 ("Data To Send")) -> (x .or. y?=w144:u8)
          n28 = Build Array(w144) -> (w163:u8[])
          n29 = call <vilib>:"WPI_I2CWrite.vi"("error in (no error)"=w150, "I2CDataToSend"=w163, "I2CRegister"=u8 35 ("Data To Send"), "I2CDevRef"=w158) -> ("error out"=w149:errorcluster, "I2CDevRef"=w155:T8)  [unwired: 6 out]
          n30 = Boolean To (0,1)(Boolean=w141) -> (0, 1=w142:i16)
          n31 = Or(x=w142, y=u8 16 ("Data To Send")) -> (x .or. y?=w140:i16)
          n32 = Build Array(w140) -> (w152:i16[])
          n33 = call <vilib>:"WPI_I2CWrite.vi"("error in (no error)"=w149, "I2CDataToSend"=w152, "I2CRegister"=u8 36 ("Data To Send"), "I2CDevRef"=w155) -> ("error out"=w148:errorcluster, "I2CDevRef"=w154:T8)  [unwired: 6 out]
          n34 = Logical Shift(y=i16 6, x=w135) -> (x << y=w137:u32)
          n35 = Or(x=w137, y=u8 15 ("Data To Send")) -> (x .or. y?=w133:u32)
          n36 = Build Array(w133) -> (w134:u32[])
          n37 = call <vilib>:"WPI_I2CWrite.vi"("error in (no error)"=w148, "I2CDataToSend"=w134, "I2CRegister"=u8 32 ("Data To Send"), "I2CDevRef"=w154) -> ("error out"=w166:errorcluster, "I2CDevRef"=w167:T8)  [unwired: 6 out]
        }
        frame Default {
          n38 = call <vilib>:"Error Cluster From Error Code.vi"("error in (no error)"=w171, "error message (\"\")"="I2C Device at this address not recognized,\ndevice is not a STMicroelectonics \nL3GD20 or L3GD20H Gyro" ("error message (\"\")"), "error code (0)"=257) -> ("error out"=w168:errorcluster)  [unwired: 6 in]
        }
      }
      n39 = Unbundle By Name(w87) -> ("DevStatus"=w86:errorcluster, "Device Address"=w85:u8, "Handle"=w78:i32, "I2C Bus"=w77:T3)
    }
  }
  n40 = disable-structure shown="Disabled" {
    frame Disabled {
      n41 = node-c288() -> (w177:T9)
      n42 = call "IMURefNum Registry Get.vi"("refnum name"="AdaFruit IMU RefNum") -> ("error out"=w173:errorcluster, "AdaIMUDevRef Out"=w174:T6)  [unwired: 9 in]
      n43 = timed-loop {
        tunnel: w174 -> [w191]
        tunnel: w173 -> [w190]
        timing: w177 -> [_]
        timing-out: [_] -> w176
        stop <- FALSE stop-if-true
        n44 = node-c288() -> (→"Late?":bool)  [unwired: 1 in]
        n45 = case shown="True" "Reset" {
          tunnel: w191 -> [w201 w205]
          tunnel: [w201 w204] -> w193
          tunnel: [w200 w203] -> w192
          tunnel: w190 -> [w200 w202]
          frame False {
          }
          frame True {
            # "Gyro"
            n46 = call "IMUReset.vi"("error in (no error)"=w202, "AdaIMUDevRef"=w205) -> ("error out"=w203:errorcluster, "AdaIMUDevRef Out"=w204:T6)  [unwired: 8 in]
          }
        }
        n47 = call "IMURead.vi"("AdaIMUDevRef"=w193, "error in"=w192) -> ("Gyro"=w188:T12, "Accel"=w187:T13, "Mag"=w186:T14)  [unwired: 9 in, 2 out]
        n48 = call "IMUComplementaryFilter.vi"("tau acc"=0.4, "tau mag"=0.1, "Gyro"=w188, "Accel"=w187, "Mag"=w186, "Tilt Comp (Yaw)"=FALSE) -> ("Roll"=→"Roll":dbl, "Pitch"=→"Pitch":dbl, "Yaw"=→"Yaw":dbl)  [unwired: 7 in]
        n49 = node-c288("Period") -> ()  [unwired: 1 out]
      }
      n50 = node-c288(w176) -> ()  [unwired: 1 out]
    }
    frame Enabled {
    }
  }
  n51 = Unbundle By Name("Accel Set") -> ("Sense Enable"=w49:bool, "HPF Enable"=w65:bool, "HPCF"=w64:enum8{"00", "01", "10", "11"}, "Range"=w56:u8, "Data Rate"=w63:T15, "Accel Scale"=w57:T16, "Motion Thresh"=w54:dbl)
  n52 = disable-structure shown="Disabled" {
    frame Disabled {
      n53 = call "IMUOpen.vi"("MagCal"=TRUE, "Accel Set"="Accel Set 2", "Mag Set"="Mag Set 2", "Gyro Set"="Gyro Set 2", "Fast"=TRUE, "CalSamples"=30 ("CalAvg"), "I2C Bus"=i2c_bus."I2C On-Board") -> ("AdaIMUDevRef Out"=w214:T6)  [unwired: 2 in, 2 out]
      n54 = call "IMURefNum Registry Set.vi"("refnum name"="AdaFruit IMU RefNum", "AdaIMUDevRef"=w214) -> ()  [unwired: 8 in, 2 out]
    }
    frame Enabled {
    }
  }
  n55 = Unbundle By Name("Mag Set") -> ("Sense Enable"=w48:bool, "Range"=w47:u8, "Data Rate"=w52:T17, "Mag Scale"=w44:T16, "Mag Offset"=w43:cluster{"Xzero":dbl, "Yzero":dbl, "Zzero":dbl}, "Anomaly Thresh"=w40:dbl, "Local Mag"=w39:dbl)
  n56 = case shown="True" w49 {
    tunnel: [u8 0 ("Device Address") w248] -> w50
    tunnel: w65 -> [_ w223]
    tunnel: w64 -> [_ w222]
    tunnel: w63 -> [_ w221]
    tunnel: w56 -> [_ w220]
    tunnel: "I2C Bus" -> [_ w219]
    frame False {
    }
    frame True {
      # "Accelerometer"
      n57 = call <vilib>:"WPI_I2COpen.vi"("Device Address"=u8 25 ("Data To Send"), "I2C Bus"=w219) -> ("I2CDevRef"=w226:T8)  [unwired: 8 in, 1 out]
      n58 = Boolean To (0,1)(Boolean=w223) -> (0, 1=w247:i16)
      n59 = Logical Shift(y=i16 4, x=w222) -> (x << y=w243:u32)
      n60 = Logical Shift(y=i16 3, x=w247) -> (x << y=w244:i16)
      n61 = Or(x=w244, y=w243) -> (x .or. y?=w227:u32)
      n62 = Build Array(w227) -> (w229:u32[])
      n63 = call <vilib>:"WPI_I2CWrite.vi"("I2CDataToSend"=w229, "I2CRegister"=u8 33 ("Data To Send"), "I2CDevRef"=w226) -> ("I2CDevRef"=w225:T8)  [unwired: 7 in, 1 out]
      n64 = Logical Shift(y=i16 4, x=w220) -> (x << y=w232:u8)
      n65 = Or(x=u8 128 ("Data To Send"), y=w232) -> (x .or. y?=w231:u8)
      n66 = Build Array(w231) -> (w235:u8[])
      n67 = call <vilib>:"WPI_I2CWrite.vi"("I2CDataToSend"=w235, "I2CRegister"=u8 35 ("Data To Send"), "I2CDevRef"=w225) -> ("I2CDevRef"=w224:T8)  [unwired: 7 in, 1 out]
      n68 = Logical Shift(y=i16 4, x=w221) -> (x << y=w238:u32)
      n69 = Or(x=w238, y=u8 7 ("Data To Send")) -> (x .or. y?=w237:u32)
      n70 = Build Array(w237) -> (w241:u32[])
      n71 = call <vilib>:"WPI_I2CWrite.vi"("I2CDataToSend"=w241, "I2CRegister"=u8 32 ("Data To Send"), "I2CDevRef"=w224) -> ("I2CDevRef"=w236:T8)  [unwired: 7 in, 1 out]
      n72 = Unbundle By Name(w236) -> ("Device Address"=w248:u8)
    }
  }
  n73 = case shown="True" w48 {
    tunnel: w47 -> [_ w269]
    tunnel: [u8 0 ("Device Address") w268] -> w55
    tunnel: w52 -> [_ w253]
    tunnel: "I2C Bus" -> [_ w251]
    frame False {
    }
    frame True {
      # "Magnetometer"
      n74 = call <vilib>:"WPI_I2COpen.vi"("Device Address"=u8 30 ("Data To Send"), "I2C Bus"=w251) -> ("I2CDevRef"=w265:T8)  [unwired: 8 in, 1 out]
      n75 = Logical Shift(y=i16 5, x=w269) -> (x << y=w255:u8)
      n76 = Build Array(w255) -> (w263:u8[])
      n77 = call <vilib>:"WPI_I2CWrite.vi"("I2CDataToSend"=w263, "I2CRegister"=u8 1 ("Data To Send"), "I2CDevRef"=w265) -> ("I2CDevRef"=w266:T8)  [unwired: 7 in, 1 out]
      n78 = Logical Shift(y=i16 2, x=w253) -> (x << y=w254:u32)
      n79 = Build Array(w254) -> (w260:u32[])
      n80 = call <vilib>:"WPI_I2CWrite.vi"("I2CDataToSend"=w260, "I2CRegister"=u8 0 ("Data To Send"), "I2CDevRef"=w266) -> ("I2CDevRef"=w267:T8)  [unwired: 7 in, 1 out]
      n81 = Build Array(i16 0 ("y")) -> (w258:i16[])
      n82 = call <vilib>:"WPI_I2CWrite.vi"("I2CDataToSend"=w258, "I2CRegister"=u8 2 ("Data To Send"), "I2CDevRef"=w267) -> ("I2CDevRef"=w259:T8)  [unwired: 7 in, 1 out]
      n83 = Unbundle By Name(w259) -> ("Device Address"=w268:u8)
    }
  }
  n84 = Bundle By Name(cluster=T6 {"DevStatus"={"status"=FALSE, "code"=0, "source"=""}, "Gyro Address"=0, "Gyro Range"=0, "Mean Rates"={"Xmo"=0.0, "Ymo"=0.0, "Zmo"=0.0}, "StdDev Rates"={"Xsdo"=0.0, "Ysdo"=0.0, "Zsdo"=0.0}, "Fast"=FALSE, "Reset"=FALSE, "Accel Address"=0, "Accel Range"=0, "Accel Scale"={"Xscale"=0.0, "Yscale"=0.0, "Zscale"=0.0}, "Mag Address"=0, "Mag Range"=0, "G Sense"=FALSE, "A Sense"=FALSE, "M Sense"=FALSE, "Accel Offset"={"Xzero"=0.0, "Yzero"=0.0, "Zzero"=0.0}, "Motion Thresh"=0.0, "Mag Scale"={"Xscale"=0.0, "Yscale"=0.0, "Zscale"=0.0}, "Mag Offset"={"Xzero"=0.0, "Yzero"=0.0, "Zzero"=0.0}, "I2C Bus"=enum."I2C On-Board", "Handle"=0, "Anomaly Thresh"=0.0, "Local Mag"=0.0} ("AdaIMUDevRef"), "G Sense"=w51, "Gyro Range"=w61, "DevStatus"=w69, "Gyro Address"=w68, "Handle"=w41, "I2C Bus"=w42, "Fast"="Fast", "A Sense"=w49, "Accel Address"=w50, "Accel Range"=w56, "Accel Scale"=w57, "Motion Thresh"=w54, "M Sense"=w48, "Mag Address"=w55, "Mag Range"=w47, "Mag Scale"=w44, "Mag Offset"=w43, "Anomaly Thresh"=w40, "Local Mag"=w39) -> (w36:T6)
  n85 = for {
    N: 8 -> [_]
    tunnel: w36 -> [w273]
    tunnel: w46 -> [w272]
    tunnel: [w271] -> w37
    tunnel: [w270] -> w45
    n86 = call "IMURead.vi"("AdaIMUDevRef"=w273, "error in"=w272) -> ("AdaIMUDevRef Out"=w271:T6, "error out"=w270:errorcluster)  [unwired: 9 in, 3 out]
    n87 = Wait (ms)(milliseconds to wait=u32 50) -> ()  [unwired: 1 out]
  }
  n88 = Initialize Array(0.0 ("element"), "CalSamples", 3 ("dimension size")) -> (w29:dbl[][])
  n89 = Initialize Array(0.0 ("element"), 3 ("dimension size")) -> (w11:dbl[])
  n90 = while "Gyro & Accelerometer Calibration" {
    tunnel: w37 -> [w297]
    tunnel: w45 -> [w310]
    tunnel: "CalSamples" -> [w305]
    tunnel: w29 -> [w304]
    tunnel: w29 -> [w300]
    tunnel: [w299] -> w22
    tunnel: [w295] -> w15
    tunnel: [w294] -> w14
    tunnel: w11 -> [w293]
    tunnel: [w277] -> w4
    tunnel: [w276] -> w3
    i -> [w275]
    stop <- w278 stop-if-true
    # "Preserve Mag Set\ncal values should\nMagnetic Cal be\nunrequested."
    # "'Zero' Gyro rate, Accelerometer,\nand Magnetometer biases\n(offsets).  Initialize Mag scale\nfactors to 1.  This allows the\nIMU Open VI to call the IMU\nRead VI and obtain raw readings\nso IMU Open can determine\ncalibration settings for the three\ndevices.\n\nNote: the Accelerometer scale\nfactors are not initialized since\nthat calibration should be\nperformed off robot, as it\nrequires the sensor to be moved\nin all 3 dimensions.  These values\nare either determined experimentally\noff-robot (to improve upon the\nstandard sensitivity values given in\nthe sensor spec sheet), or assumed\nto be a value of one for each axis."
    # "Report Bad Calibration if any\naxis Standard Deviation is too\nhigh.  This is caused by movement\nduring the cal period, insufficient\nwarmup time, or possibly bad\nsensor.  Thresholds were\ndetermined experimentally."
    # "If BadCal, try one\nmore time."
    # "Read a sample set of measurements\nfrom each axis for Gyro and Accelerometer\ncalibration.  Sample size determined by\nCalSamples parameter.  The intent is to\ndetermine the Gyro rate and Accelerometer\noutputs under the condition that the \nsensor is not moving, in order to identify\na 'zero' rate reference for the Gyro and the\nbiases (offsets from zero) for the Accel.\nMagnetometer calibration is performed next\n(if MagCal selected True), since this requires\nthe sensor to be moving as data is collected."
    # "Determine zero (rate) reference\n(dataset mean) for each axis, and\nevaluate level of variation\n(dataset standard deviation)\nto assess quality of calibration."
    n91 = flat-sequence {
      tunnel: w297 -> [w333]
      tunnel: [w333] -> w296
      tunnel: [w332] -> w295
      tunnel: [w331] -> w294
      tunnel: [w338] -> w298
      tunnel: w296 -> [w337]
      frame #0 {
        n92 = Unbundle By Name(w333) -> ("Mag Scale"=w332:T16, "Mag Offset"=w331:cluster{"Xzero":dbl, "Yzero":dbl, "Zzero":dbl})
      }
      frame #1 {
        w335 = T18 {"Accel Zero.Zzero"=0.0, "Accel Zero.Zzero 2"=0.0, "Accel Zero.Zzero 3"=0.0}
        n93 = Bundle By Name(cluster=w337, "Mean Rates"=w335, "Accel Offset"=T18 {"Accel Zero.Zzero"=0.0, "Accel Zero.Zzero 2"=0.0, "Accel Zero.Zzero 3"=1.0}, "Mag Offset"=w335, "Mag Scale"=T18 {"Accel Zero.Zzero"=1.0, "Accel Zero.Zzero 2"=1.0, "Accel Zero.Zzero 3"=1.0}) -> (w338:T6)
      }
    }
    n94 = node-c288(i64 30 ("Period"), 200 ("Priority")) -> (w330:T9)  [unwired: 1 in]
    n95 = timed-loop "Generate Accel & Gyro Dataset" {
      tunnel: w310 -> [w353]
      tunnel: w298 -> [w354]
      timing: w330 -> [_]
      timing-out: [_] -> w329
      tunnel: w304 -> [w350]
      tunnel: [w357] -> w324
      tunnel: [w359] -> w311
      tunnel: [w358] -> w328
      tunnel: w305 -> [w355]
      tunnel: [w349] -> w285
      tunnel: w300 -> [w348]
      tunnel: w293 -> [w345]
      i -> [w339]
      stop <- w360 stop-if-true
      n96 = Decrement(x=w355) -> (x-1=w352:i32)
      n97 = call "IMURead.vi"("AdaIMUDevRef"=w354, "error in"=w353) -> ("AdaIMUDevRef Out"=w359:T6, "Gyro"=w347:T12, "Accel"=w341:T13, "error out"=w358:errorcluster)  [unwired: 9 in, 1 out]
      n98 = Equal?(x=w352, y=w339) -> (x = y?=w360:bool)
      n99 = Unbundle By Name(w341) -> ("Xaccel"=w343:dbl, "Yaccel"=w342:dbl, "Zaccel"=w340:dbl)
      n100 = Cluster To Array(cluster=w347) -> (array=w346:dbl[])
      n101 = Replace Array Subset(array=w345, new element #1=w343, new element #2=w342, new element #3=w340) -> (w344:dbl[])  [unwired: 3 in]
      n102 = feedback #1(w350) -> (w356:dbl[][])
      n103 = Replace Array Subset(array=w356, new element=w346, index (row)=w339) -> (w357:dbl[][])  [unwired: 1 in]
      n104 = feedback-in #1(w357) -> ()
      n105 = feedback #2(w348) -> (w351:dbl[][])
      n106 = Replace Array Subset(array=w351, new element=w344, index (row)=w339) -> (w349:dbl[][])  [unwired: 1 in]
      n107 = feedback-in #2(w349) -> ()
    }
    "error out" <- w328
    n108 = node-c288(w329) -> ()  [unwired: 1 out]
    n109 = Index Array(array=w285, index (col)=0 ("index")) -> (element=w286:dbl[])  [unwired: 1 in]
    n110 = Index Array(array=w285, index (col)=1 ("index")) -> (element=w287:dbl[])  [unwired: 1 in]
    n111 = Index Array(array=w285, index (col)=2 ("index")) -> (element=w288:dbl[])  [unwired: 1 in]
    n112 = call <vilib>:"Std Deviation and Variance.vi"("X"=w286) -> ("mean"=w284:dbl, "standard deviation"=w281:dbl)  [unwired: 1 in, 1 out]
    n113 = call <vilib>:"Std Deviation and Variance.vi"("X"=w287) -> ("mean"=w283:dbl, "standard deviation"=w280:dbl)  [unwired: 1 in, 1 out]
    n114 = call <vilib>:"Std Deviation and Variance.vi"("X"=w288) -> ("mean"=w282:dbl, "standard deviation"=w279:dbl)  [unwired: 1 in, 1 out]
    n115 = Index Array(array=w324, index (col)=0 ("index")) -> (element=w327:dbl[])  [unwired: 1 in]
    n116 = Index Array(array=w324, index (col)=1 ("index")) -> (element=w326:dbl[])  [unwired: 1 in]
    n117 = Index Array(array=w324, index (col)=2 ("index")) -> (element=w325:dbl[])  [unwired: 1 in]
    n118 = call <vilib>:"Std Deviation and Variance.vi"("X"=w327) -> ("mean"=w319:dbl, "standard deviation"=w315:dbl)  [unwired: 1 in, 1 out]
    n119 = call <vilib>:"Std Deviation and Variance.vi"("X"=w326) -> ("mean"=w318:dbl, "standard deviation"=w292:dbl)  [unwired: 1 in, 1 out]
    n120 = call <vilib>:"Std Deviation and Variance.vi"("X"=w325) -> ("mean"=w317:dbl, "standard deviation"=w314:dbl)  [unwired: 1 in, 1 out]
    n121 = Max & Min(x=w280, y=w279) -> (max(x,y)=w301:dbl)  [unwired: 1 out]
    n122 = Max & Min(x=w281, y=w301) -> (max(x,y)=w302:dbl)  [unwired: 1 out]
    n123 = Greater?(x=w302, y=0.03) -> (0:w276:bool)
    n124 = Max & Min(x=w292, y=w314) -> (max(x,y)=w316:dbl)  [unwired: 1 out]
    n125 = Max & Min(x=w315, y=w316) -> (max(x,y)=w313:dbl)  [unwired: 1 out]
    n126 = Bundle By Name(cluster=w311, "Mean Rates.Xmo"=w319, "StdDev Rates.Xsdo"=w315, "Mean Rates.Ymo"=w318, "StdDev Rates.Ysdo"=w292, "Mean Rates.Zmo"=w317, "StdDev Rates.Zsdo"=w314, "Accel Offset.Xzero"=w284, "Accel Offset.Yzero"=w283, "Accel Offset.Zzero"=w282) -> (w299:T6)
    n127 = Greater?(x=w313, y=0.5) -> (0:w277:bool)
    n128 = Equal?(x=1, y=w275) -> (x = y?=w309:bool)
    n129 = Not(x=w277) -> (.not. x?=w307:bool)
    n130 = Or(x=w307, y=w309) -> (x .or. y?=w278:bool)
  }
  n131 = Bundle By Name(cluster=T1 {"BadCal Gyro"=FALSE, "BadCal Accel"=FALSE, "BadCal Mag"=FALSE} ("Cal Status"), "BadCal Gyro"=w4, "BadCal Accel"=w3) -> (w1:T1)
  n132 = case shown="True" "MagCal" {
    selector: "MagCal" -> [w369 w372]
    tunnel: [w369 w372] -> w19
    tunnel: [w370 w374] -> w21
    tunnel: w22 -> [w370 w374]
    frame False {
      n133 = local write "stop loop"(TRUE ("true")) -> ()
    }
    frame True {
      n134 = One Button Dialog(message="Rotate robot 360 deg in horizontal plane.\nBest data results from rotating about \nactual sensor axis.\n\nSelect OK to begin data collection.") -> ()  [unwired: 1 in, 1 out]
      "stop loop" <- FALSE ("true")
    }
  }
  n135 = case shown="True" w19 {
    frame False {
    }
    frame True {
      n136 = One Button Dialog(message="Select OK when\nrotation is complete.") -> (true=w375:bool)  [unwired: 1 in]
      n137 = local write "stop loop"(w375) -> ()
    }
  }
  n138 = node-c288(i64 30 ("Period"), 200 ("Priority")) -> (w34:T9)  [unwired: 1 in]
  n139 = Initialize Array(0.0 ("element"), 3 ("dimension size")) -> (w8:dbl[])
  n140 = Initialize Array(0.0 ("element"), 0 ("Samples"), 3 ("dimension size")) -> (w24:dbl[][])
  n141 = timed-loop "Generate Magnetometer Dataset" {
    timing: w34 -> [_]
    timing-out: [_] -> w33
    tunnel: [w384] -> w17
    tunnel: [w382] -> w18
    tunnel: w24 -> [w381]
    tunnel: w19 -> [w379]
    tunnel: w21 -> [w380]
    tunnel: [w379] -> w16
    tunnel: w8 -> [w377]
    i -> [w383]
    stop <- w378 stop-if-true
    # "Gather Mag data as Robot is rotated in X-Y plane."
    n142 = local read "stop loop"() -> (w378:bool)
    n143 = case shown="True" w379 {
      tunnel: [w386 w398] -> w384
      tunnel: w383 -> [_ w396]
      tunnel: [w385 w395] -> w382
      tunnel: w381 -> [w385 w394]
      tunnel: w380 -> [w386 w393]
      tunnel: w377 -> [_ w388]
      frame False {
      }
      frame True {
        n144 = call "IMURead.vi"("AdaIMUDevRef"=w393) -> ("AdaIMUDevRef Out"=w398:T6, "Mag"=w391:T14)  [unwired: 10 in, 3 out]
        n145 = Unbundle By Name(w391) -> ("Xmag"=w390:dbl, "Ymag"=w392:dbl, "Zmag"=w389:dbl)
        n146 = Replace Array Subset(array=w388, new element #1=w390, new element #2=w392, new element #3=w389) -> (w387:dbl[])  [unwired: 3 in]
        n147 = feedback #3(w394) -> (w397:dbl[][])
        n148 = Insert Into Array(array=w397, index (row)=w396, new element=w387) -> (w395:dbl[][])  [unwired: 1 in]
        n149 = feedback-in #3(w395) -> ()
      }
    }
  }
  n150 = node-c288(w33) -> ()  [unwired: 1 out]
  n151 = case "Magnetometer Calibration" shown="True" w16 {
    tunnel: w18 -> [_ w433]
    tunnel: w17 -> [w405 w439]
    tunnel: [w404 w438] -> w7
    tunnel: w15 -> [w403 _]
    tunnel: w14 -> [w402 _]
    tunnel: [FALSE w411] -> w5
    frame False {
      # "If not calibrating Magnetometer, use calibration settings\nprovided to IMU Open within Mag Set cluster."
      n152 = Bundle By Name(cluster=w405, "Mag Scale"=w403, "Mag Offset"=w402) -> (w404:T6)
    }
    frame True {
      (unwired) path "C:/tmp/Mag_data.csv" ("file path (dialog if empty)")
      w443 = 1.0 ("y")
      w440 = 2.0 ("y")
      # "Biaxial"
      # "Triaxial"
      # "cRIO address format"
      # "Store mag data to roboRIO for review"
      # "Report Bad Calibration if any magnetic\nvector magnitude is too different from\nEarth field.  This is caused by on-Robot\nSoft Iron, near-by off-Robot Hard Iron,\nor possibly bad sensor.  Threshold was\ndetermined experimentally."
      # "Z values"
      # "Y values"
      # "X values"
      # "Ref http://www.cypress.com/?docID=49962\neqs 38-43 (and correcting for typo in eq 43)\nfor simple calibration of Magnetometer\n(in 2D X-Y plane only)."
      n153 = Index Array(array=w433, index (col)=0 ("index (row)")) -> (element=w424:dbl[])  [unwired: 1 in]
      n154 = Index Array(array=w433, index (col)=1 ("index (row)")) -> (element=w423:dbl[])  [unwired: 1 in]
      n155 = Bundle(w424, w423) -> (→"XY Mag":cluster{dbl[], dbl[]})  [unwired: 1 in]
      n156 = call-poly <vilib>:"Write To Spreadsheet File.vi"("delimiter (\\t)"="," ("delimiter (\\t)"), "2D data"=w433, "file path (dialog if empty)"=path "/home/lvuser/Mag_data.csv") -> ()  [unwired: 5 in, 1 out]
      n157 = Index Array(array=w433, index (col)=2 ("index (row)")) -> (element=w422:dbl[])  [unwired: 1 in]
      n158 = Array Max & Min(array=w424) -> (max value=w449:dbl, min value=w448:dbl)  [unwired: 2 out]
      n159 = Array Max & Min(array=w423) -> (max value=w452:dbl, min value=w451:dbl)  [unwired: 2 out]
      n160 = Add(x=w449, y=w448) -> (x+y=w450:dbl)
      n161 = Subtract(x=w449, y=w448) -> (x-y=w446:dbl)
      n162 = Add(x=w452, y=w451) -> (x+y=w453:dbl)
      n163 = Subtract(x=w452, y=w451) -> (x-y=w447:dbl)
      n164 = Divide(x=w450, y=w440) -> (x/y=w442:dbl)
      n165 = Divide(x=w453, y=w440) -> (x/y=w441:dbl)
      n166 = Divide(x=w447, y=w446) -> (x/y=w445:dbl)
      n167 = Reciprocal(x=w445) -> (1/x=w444:dbl)
      n168 = Max & Min(x=w445, y=w443) -> (max(x,y)=w418:dbl)  [unwired: 1 out]
      "Xmagscale" <- w418
      n169 = Max & Min(x=w443, y=w444) -> (max(x,y)=w421:dbl)  [unwired: 1 out]
      "Ymagscale" <- w421
      n170 = Multiply(x=w442, y=w418) -> (x*y=w420:dbl)
      "Xmagzero" <- w420
      n171 = Multiply(x=w441, y=w421) -> (x*y=w419:dbl)
      "Ymagzero" <- w419
      n172 = Array Size(array=w424) -> (size(s)=w432:i32)
      n173 = for {
        N: w432 -> [_]
        tunnel: w424 -> [w463] mode=indexing
        tunnel: w423 -> [w460] mode=indexing
        tunnel: w422 -> [w471] mode=indexing
        tunnel: [w470] -> w431 mode=indexing
        tunnel: [w466] -> w410 mode=indexing
        tunnel: w418 -> [w464]
        tunnel: w421 -> [w459]
        tunnel: w420 -> [w462]
        tunnel: w419 -> [w458]
        tunnel: [w457] -> w415 mode=indexing
        tunnel: [w456] -> w414 mode=indexing
        # "Root-Sum-Square"
        n174 = Multiply(x=w463, y=w464) -> (x*y=w465:dbl)
        n175 = Multiply(x=w460, y=w459) -> (x*y=w461:dbl)
        n176 = Subtract(x=w465, y=w462) -> (x-y=w457:dbl)
        n177 = Subtract(x=w461, y=w458) -> (x-y=w456:dbl)
        n178 = Square(x=w463) -> (x^2=w472:dbl)
        n179 = Square(x=w460) -> (x^2=w473:dbl)
        n180 = Square(x=w471) -> (x^2=w474:dbl)
        n181 = Square(x=w457) -> (x^2=w469:dbl)
        n182 = Square(x=w456) -> (x^2=w468:dbl)
        n183 = Compound Arithmetic op=ADD(w472, w473, w474) -> (w475:dbl)
        n184 = Compound Arithmetic op=ADD(w469, w468) -> (w467:dbl)
        n185 = Square Root(x=w475) -> (sqrt(x)=w470:dbl)
        n186 = Square Root(x=w467) -> (sqrt(x)=w466:dbl)
      }
      n187 = Bundle By Name(cluster=w439, "Mag Offset.Xzero"=w420, "Mag Offset.Yzero"=w419, "Mag Offset.Zzero"=0.0, "Mag Scale.Xscale"=w418, "Mag Scale.Yscale"=w421, "Mag Scale.Zscale"=1.0) -> (w438:T6)
      n188 = Array Max & Min(array=w431) -> (max value=w430:dbl, min value=w426:dbl)  [unwired: 2 out]
      n189 = call <vilib>:"Std Deviation and Variance.vi"("X"=w410) -> ("mean"=→"Local Magnitude (uT)":dbl, "standard deviation"=w408:dbl)  [unwired: 1 in, 1 out]
      n190 = Bundle(w415, w414) -> (→"XY Mag, Cal'd":cluster{dbl[], dbl[]})  [unwired: 1 in]
      n191 = Subtract(x=w430, y=w426) -> (x-y=w429:dbl)
      n192 = Multiply(x=w408, y=3.0) -> (x*y=w406:dbl)
      "Anomaly Tol (uT)" <- w406
      n193 = Divide(x=w429, y=2.0) -> (x/y=w427:dbl)
      "Half-Range" <- w427
      n194 = Greater?(x=w406, y=4.0) -> (0:w411:bool)
      n195 = Add(x=w427, y=w426) -> (x+y=→"Mid-Pnt":dbl)
    }
  }
  "AdaIMUDevRef Out" <- w7
  n196 = Bundle By Name(cluster=w1, "BadCal Mag"=w5) -> (→"Cal Result":T1)
